vi "Input 信息提取.vi"(11 "输入读取":T1) -> (2 "输入读取信号":string[](array[string]))   [LabVIEW 2017]
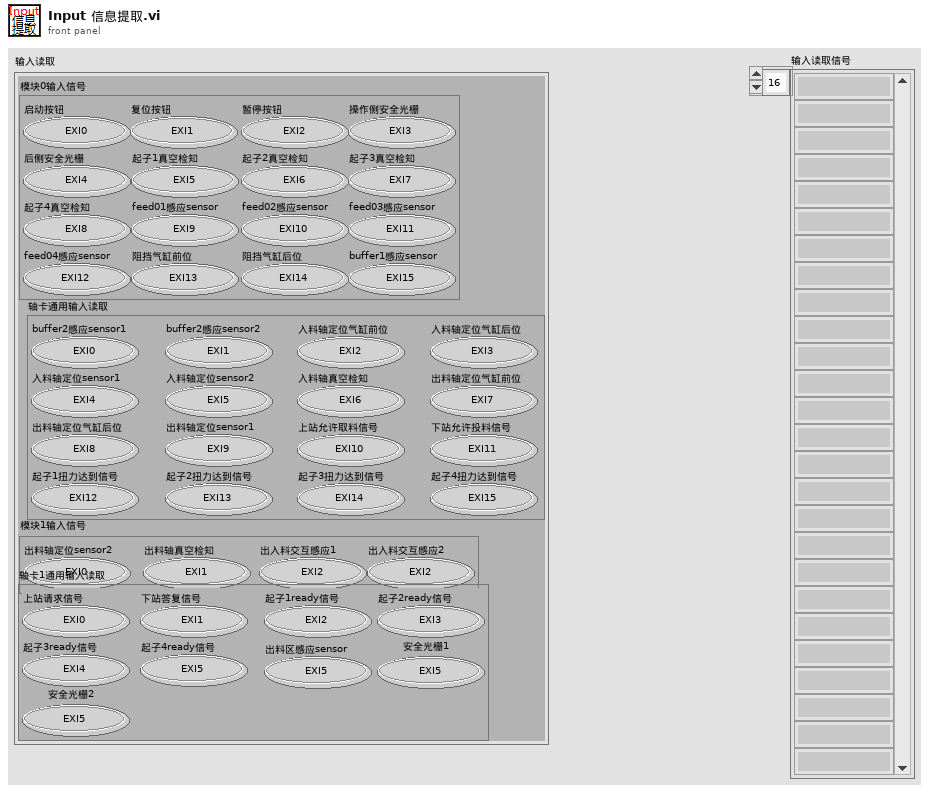
[diagram p1: front panel]
types:
  T1 = typedef "输入读取.ctl" = cluster{"模块0输入信号":T2, "轴卡通用输入读取":T3, "模块1输入信号":T4, "轴卡1通用输入读取":T5}
  T2 = typedef "模块0输入读取.ctl" = cluster{"启动按钮":bool, "复位按钮":bool, "暂停按钮":bool, "操作侧安全光栅":bool, "后侧安全光栅":bool, "起子1真空检知":bool, "起子2真空检知":bool, "起子3真空检知":bool, "起子4真空检知":bool, "feed01感应sensor":bool, "feed02感应sensor":bool, "feed03感应sensor":bool, "feed04感应sensor":bool, "阻挡气缸前位":bool, "阻挡气缸后位":bool, "buffer1感应sensor":bool}
  T3 = typedef "轴卡0通用输入读取.ctl" = cluster{"buffer2感应sensor1":bool, "buffer2感应sensor2":bool, "入料轴定位气缸前位":bool, "入料轴定位气缸后位":bool, "入料轴定位sensor1":bool, "入料轴定位sensor2":bool, "入料轴真空检知":bool, "出料轴定位气缸前位":bool, "出料轴定位气缸后位":bool, "出料轴定位sensor1":bool, "上站允许取料信号":bool, "下站允许投料信号":bool, "起子1扭力达到信号":bool, "起子2扭力达到信号":bool, "起子3扭力达到信号":bool, "起子4扭力达到信号":bool}
  T4 = typedef "模块1输入读取.ctl" = cluster{"出料轴定位sensor2":bool, "出料轴真空检知":bool, "出入料交互感应1":bool, "出入料交互感应2":bool}
  T5 = typedef "轴卡1通用输入读取.ctl" = cluster{"上站请求信号":bool, "下站答复信号":bool, "起子1ready信号":bool, "起子2ready信号":bool, "起子3ready信号":bool, "起子4ready信号":bool, "出料区感应sensor":bool, "安全光栅1":bool, "安全光栅2":bool}
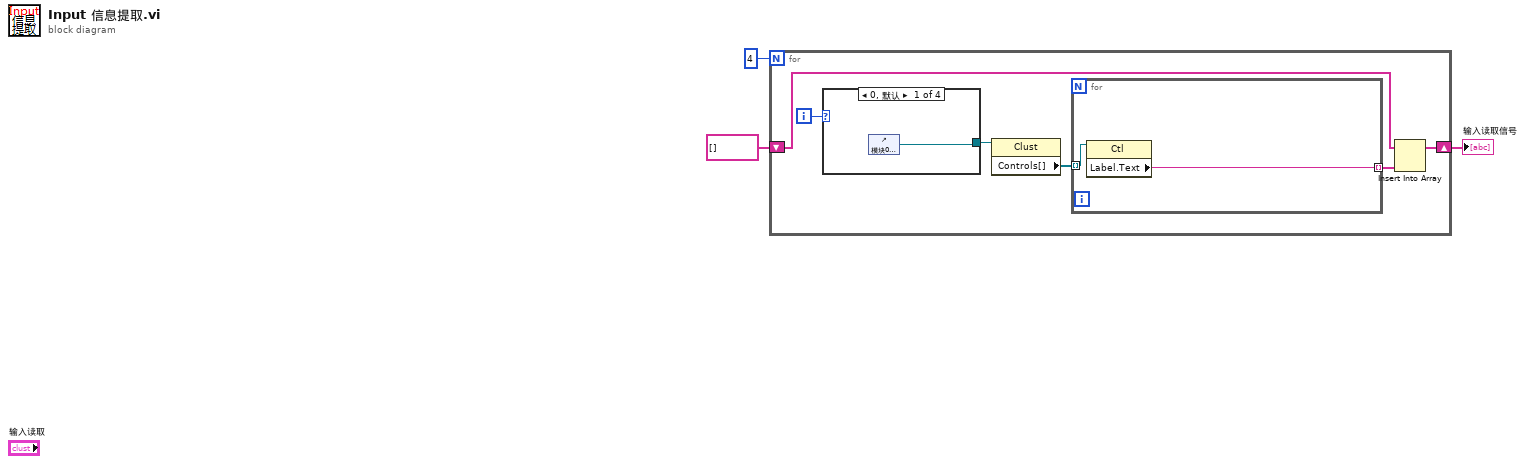
[diagram p0: block diagram]
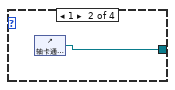
[diagram p2: hidden frame]
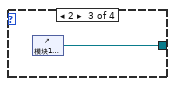
[diagram p3: hidden frame]
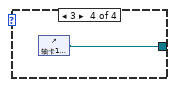
[diagram p4: hidden frame]
diagram:
  n1 = for {
    N: 4 -> [_]
    shift-right: [w6] -> w1
    shift-left: string[] [] -> [w4]
    i -> [w9]
    n2 = case shown="0, 默认" w9 {
      tunnel: [w12 w13 w14 w15] -> w7
      frame 0, Default {
        n3 = control-ref of="模块0输入信号"() -> (w12:refnum<vi>)
      }
      frame 1 {
        n4 = control-ref of="轴卡通用输入读取"() -> (w13:refnum<vi>)
      }
      frame 2 {
        n5 = control-ref of="模块1输入信号"() -> (w14:refnum<vi>)
      }
      frame 3 {
        n6 = control-ref of="轴卡1通用输入读取"() -> (w15:refnum<vi>)
      }
    }
    n7 = property class="Clust"(reference=w7) -> ("Controls[]"=w8:refnum<vi>[])  [unwired: 1 in, 2 out]
    n8 = for {
      tunnel: w8 -> [w11] mode=indexing
      tunnel: [w10] -> w5 mode=indexing
      n9 = property class="Ctl"(reference=w11) -> ("Label.Text"=w10:string)  [unwired: 1 in, 2 out]
    }
    n10 = Insert Into Array(array=w4, new element=w5) -> (w6:string[])  [unwired: 1 in]
  }
  "输入读取信号" <- w1
